vi "myXi_InitializeFreeRunnin.vi"(7 "subimage IN":refnum<vi>, 8 "error in (no error)":errorcluster, 11 "xiCam IN":refnum<k24>) -> (0 "error out":errorcluster, 2 "Array":u8[](array[numeric]), 3 "xiCam Out":refnum<k24>)   [LabVIEW 2018]
uses:
  C:/XIMEA/API/x64/xiApi.NETX64.dll
  VisionLibrariesXimea/xiLib/xiLIB_64bit/xiLIB/xiCamLib/xiCam/PRM/PRM/PRM_v2.ctl
  VisionLibrariesXimea/xiLib/xiLIB_64bit/xiLIB/xiCamLib/xiCam/PRM/TRG_SOURCE/TRG_SOURCE.ctl
  VisionLibrariesXimea/xiLib/xiLIB_64bit/xiLIB/xiCamLib/xiCam/PRM/TRG_SELECTOR/TRG_SELECTOR.ctl
  VisionLibrariesXimea/xiLib/xiLIB_64bit/xiLIB/xiCamLib/xiLIB/xiLIB - GetPRM_INFO.vi
  VisionLibrariesXimea/xiLib/xiLIB_64bit/xiLIB/xiCamLib/xiCam/Methods/xiCam - GetParam_Float.vi
  VisionLibrariesXimea/xiLib/xiLIB_64bit/xiLIB/xiCamLib/xiCam/Methods/xiCam - GetParam_String.vi
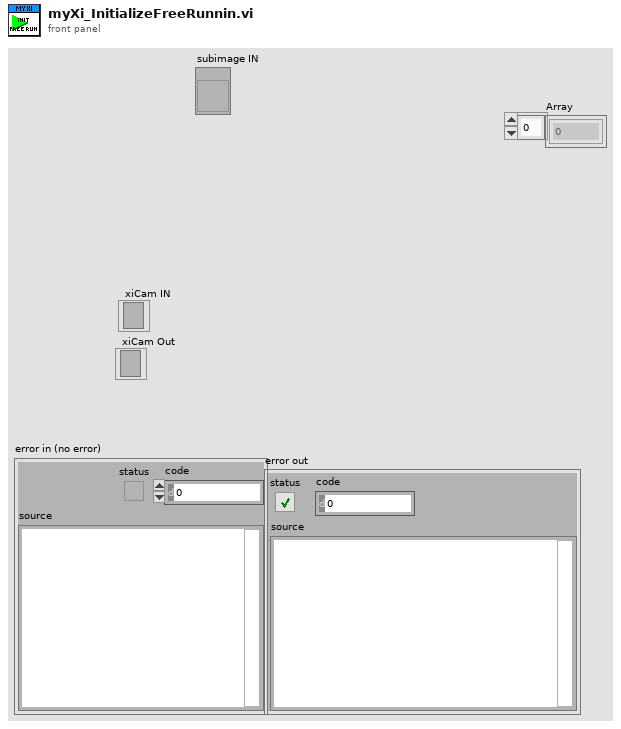
[diagram p1: front panel]
types:
  T1 = typedef "PRM_v2.ctl" = enum16{"ACQ_BUFFER_SIZE", "ACQ_FRAME_BURST_COUNT", "ACQ_TIMING_MODE", "ACQ_TRANSPORT_BUFFER_SIZE", "AE_MAX_LIMIT", "AEAG", "AEAG_LEVEL", "API_VERSION", "AG_MAX_LIMIT", "APPLY_CMS", "AUTO_BANDWIDTH_CALCULATION", "AUTO_WB", "AVAILABLE_BANDWIDTH", "AVAILABLE_BANDWIDTH_MAX", "AVAILABLE_BANDWIDTH_MIN", "BPC", "BUFFER_POLICY", "BUFFERS_QUEUE_SIZE", "CC_MATRIX_00", "CC_MATRIX_01", "CC_MATRIX_02", "CC_MATRIX_03", "CC_MATRIX_10", "CC_MATRIX_11", "CC_MATRIX_12", "CC_MATRIX_13", "CC_MATRIX_20", "CC_MATRIX_21", "CC_MATRIX_22", "CC_MATRIX_23", "CC_MATRIX_30", "CC_MATRIX_31", "CC_MATRIX_32", "CC_MATRIX_33", "CHIP_TEMP", "CMS", "COLOR_FILTER_ARRAY", "COOLING", "DEBOUNCE_EN", "DEBOUNCE_POL", "DEBOUNCE_T0", "DEBOUNCE_T1", "DEBUG_LEVEL", "DEFAULT_CC_MATRIX", "DEVICE_INSTANCE_PATH", "DEVICE_MODEL_ID", "DEVICE_NAME", "DEVICE_SN", "DEVICE_TYPE", "DEVICE_USER_ID", "DOWNSAMPLING", "DOWNSAMPLING_MAX", "DOWNSAMPLING_MIN", "DOWNSAMPLING_TYPE", "DRV_VERSION", "EXP_PRIORITY", "EXPOSURE", "EXPOSURE_DIRECT_UPDATE", "EXPOSURE_MAX", "EXPOSURE_MIN", "FFS_FILE_NAME", "FPGA1_VERSION", "FRAMERATE", "FRAMERATE_MAX", "FRAMERATE_MIN", "FREE_FFS_SIZE", "GAIN", "GAIN_DIRECT_UPDATE", "GAIN_MAX", "GAIN_MIN", "GAMMAC", "GAMMAY", "GPI_LEVEL", "GPI_MODE", "GPI_SELECTOR", "GPI_SELECTOR_MAX", "GPI_SELECTOR_MIN", "GPO_MODE", "GPO_SELECTOR", "GPO_SELECTOR_MAX", "GPO_SELECTOR_MIN", "HDR", "HDR_T1", "HDR_T2", "HEIGHT", "HEIGHT_MAX", "HEIGHT_MIN", "HOUSE_TEMP", "IMAGE_DATA_FORMAT", "IMAGE_IS_COLOR", "INPUT_CMS_PROFILE", "IS_COOLED", "IS_DEVICE_EXIST", "KNEEPOINT1", "KNEEPOINT2", "LED_MODE", "LED_SELECTOR", "LED_SELECTOR_MAX", "LED_SELECTOR_MIN", "LIMIT_BANDWIDTH", "LIMIT_BANDWIDTH_MAX", "LIMIT_BANDWIDTH_MIN", "LUT_EN", "LUT_INDEX", "LUT_INDEX_MAX", "LUT_INDEX_MIN", "LUT_VALUE", "LUT_VALUE_MAX", "LUT_VALUE_MIN", "MANUAL_WB", "MCU1_VERSION", "MCU2_VERSION", "OFFSET_X", "OFFSET_X_MAX", "OFFSET_X_MIN", "OFFSET_Y", "OFFSET_Y_MAX", "OFFSET_Y_MIN", "OUTPUT_CMS_PROFILE", "OUTPUT_DATA_BIT_DEPTH", "OUTPUT_DATA_PACKING", "READ_FILE_FFS", "RECENT_FRAME", "SENSOR_DATA_BIT_DEPTH", "SENSOR_MODE", "SENSOR_TAPS", "SHARPNESS", "SHUTTER_TYPE", "TARGET_TEMP", "TRG_DELAY", "TRG_SELECTOR", "TRG_SOFTWARE", "TRG_SOURCE", "USED_FFS_SIZE", "WB_KB", "WB_KG", "WB_KR", "WIDTH", "WIDTH_MAX", "WIDTH_MIN", "WRITE_FILE_FFS", "ACQ_BUFFER_SIZE_UNIT", "ACQ_TRANSPORT_BUFFER_COMMIT", "AEAG_ROI_HEIGHT", "AEAG_ROI_OFFSET_X", "AEAG_ROU_OFFSET_Y", "AEAG_ROI_WIDTH", "API_CONTEXT_LIST", "BINNING_HORIZONTAL", "BINNING_SELECTOR", "BINNING_VERTICAL", "COLUMN_FPN_CORRECTION", "COUNTER_SELECTOR", "COUNTER_VALUE", "DECIMATION_HORIZONTAL", "DECIMATION_SELECTOR", "DECIMATION_VERTICAL", "DEVICE_ID", "DEVICE_LOCATION_PATH", "DEVICE_MANIFEST", "DEVICE_RESET", "DEVICE_SENS_SN", "EXPOSURE_BURST_COUNT", "FFS_ACCESS_KEY", "GAIN_SELECTOR", "HW_REVISION", "IMAGE_BLACK_LEVEL", "IMAGE_DATA_BIT_DEPTH", "IMAGE_DATA_FORMAT_RGB32_ALPHA", "IMAGE_PAYLOAD_SIZE", "LENS_APERTURE_VALUE", "LENS_FEATURE", "LENS_FEATURE_SELECTOR", "LENS_FOCAL_LENGTH", "LENS_FOCUS_DISTANCE", "LENS_FOCUS_MOVE", "LENS_FOCUS_MOVEMENT_VALUE", "LENS_MODE", "OUTPUT_DATA_PACKING_TYPE", "SENSOR_CLOCK_FREQ_HZ", "SENSOR_CLOCK_FREQ_INDEX", "SENSOR_FEATURE_SELECTOR", "SENSOR_FEATURE_VALUE", "SENSOR_OUTPUT_CHANNEL_COUNT", "TRANSPORT_PIXEL_FORMAT", "TS_RST_MODE", "TS_RST_SOURCE"}
  T2 = typedef "TRG_SOURCE.ctl" = enum16{"OFF", "EDGE_RISING", "EDGE_FALLING", "SOFTWARE"}
  T3 = typedef "TRG_SELECTOR.ctl" = enum16{"FRAME_START", "EXPOSURE_ACTIVE", "FRAME_BURST_START", "FRAME_BURST_ACTIVE"}
  T4 = typedef "LVPointDoubleTypeDef.ctl" = cluster{"X":dbl, "Y":dbl}
  T5 = cluster{"2^n : x":i8, "2^n : y":i8, "lower left box Position":T4, "Height":i32, "Width":i32}
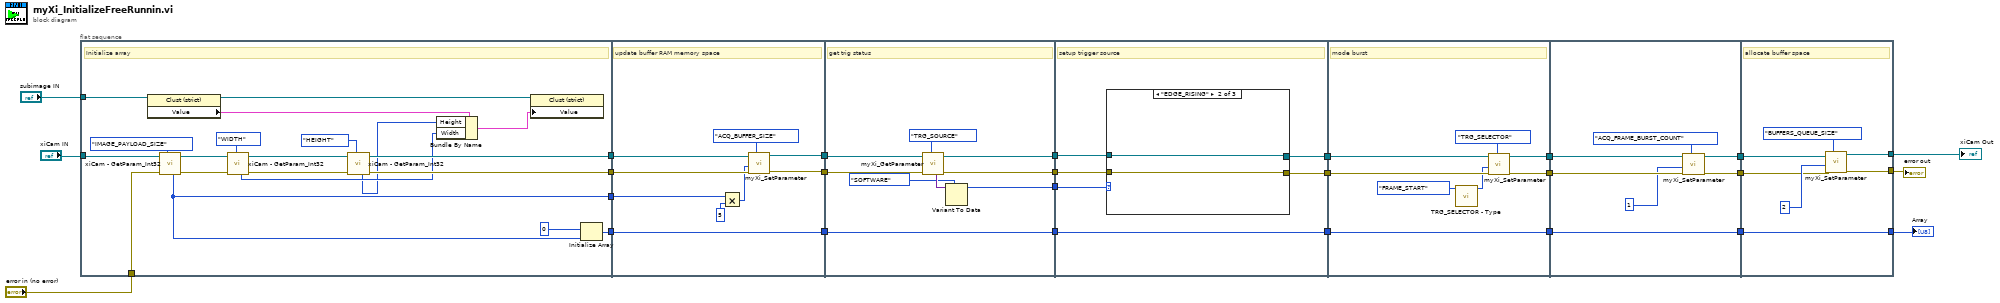
[diagram p0: block diagram]
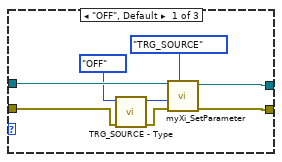
[diagram p2: hidden frame]
diagram:
  n1 = flat-sequence {
    tunnel: "xiCam IN" -> [w46]
    tunnel: [w43] -> w26
    tunnel: "error in (no error)" -> [w42]
    tunnel: [w41] -> w25
    tunnel: [w39] -> w24
    tunnel: "subimage IN" -> [w38]
    tunnel: [w27] -> w1
    tunnel: w26 -> [w53]
    tunnel: [w52] -> w23
    tunnel: w25 -> [w55]
    tunnel: [w54] -> w22
    tunnel: w24 -> [w50]
    tunnel: [w50] -> w21
    tunnel: w1 -> [w47]
    tunnel: w23 -> [w61]
    tunnel: [w60] -> w20
    tunnel: w22 -> [w63]
    tunnel: [w62] -> w19
    tunnel: w21 -> [w64]
    tunnel: [w64] -> w18
    tunnel: [w56] -> w17
    tunnel: [w69] -> w16
    tunnel: [w68] -> w15
    tunnel: w20 -> [w70]
    tunnel: w19 -> [w67]
    tunnel: [w66] -> w14
    tunnel: w18 -> [w66]
    tunnel: w17 -> [w65]
    tunnel: w16 -> [w89]
    tunnel: w15 -> [w88]
    tunnel: w14 -> [w83]
    tunnel: [w85] -> w8
    tunnel: [w84] -> w6
    tunnel: [w83] -> w4
    tunnel: w8 -> [w95]
    tunnel: [w94] -> w7
    tunnel: w6 -> [w93]
    tunnel: [w92] -> w5
    tunnel: w4 -> [w97]
    tunnel: [w97] -> w3
    tunnel: [w103] -> w11
    tunnel: [w102] -> w12
    tunnel: w7 -> [w100]
    tunnel: w5 -> [w99]
    tunnel: [w98] -> w9
    tunnel: w3 -> [w98]
    frame #0 {
      # "Initialize array"
      n2 = property class="Clust (strict)"(reference=w38) -> (reference out=w37:refnum<vi>, "Value"=w36:T5)  [unwired: 1 in, 1 out]
      n3 = call "xiCam - GetParam_Int32.vi"("PRM"=PRM_v2."IMAGE_PAYLOAD_SIZE", "error in (no error)"=w42, "xiCam In"=w46) -> ("error out"=w34:errorcluster, "xiCam Out"=w32:refnum<k24>, "Int32_Value"=w27:i32)  [unwired: 6 in]
      n4 = call "xiCam - GetParam_Int32.vi"("PRM"=PRM_v2."WIDTH", "error in (no error)"=w34, "xiCam In"=w32) -> ("error out"=w33:errorcluster, "xiCam Out"=w31:refnum<k24>, "Int32_Value"=w29:i32)  [unwired: 6 in]
      n5 = call "xiCam - GetParam_Int32.vi"("PRM"=PRM_v2."HEIGHT", "error in (no error)"=w33, "xiCam In"=w31) -> ("error out"=w41:errorcluster, "xiCam Out"=w43:refnum<k24>, "Int32_Value"=w28:i32)  [unwired: 6 in]
      n6 = Bundle By Name(cluster=w36, "Height"=w28, "Width"=w29) -> (w35:T5)
      n7 = property class="Clust (strict)"(reference=w37, "Value"=w35) -> ()  [unwired: 1 in, 2 out]
      n8 = Initialize Array "Initialize Array"(u8 0 ("element"), w27) -> (w39:u8[])
    }
    frame #1 {
      # "update buffer RAM memory space"
      n9 = Multiply(x=w47, y=i64 5 ("image frames")) -> (x*y=w49:i64)
      n10 = call "myXi_SetParameter.vi"("input PRM"=PRM_v2."ACQ_BUFFER_SIZE", "error in"=w55, "input value I32"=w49, "xiCam IN"=w53) -> ("error out"=w54:errorcluster, "xiCam Out"=w52:refnum<k24>)  [unwired: 6 in]
    }
    frame #2 {
      # "get trig status"
      n11 = call "myXi_GetParameter.vi"("input PRM"=PRM_v2."TRG_SOURCE", "error in"=w63, "xiCam IN"=w61) -> ("error out"=w62:errorcluster, "xiCam Out"=w60:refnum<k24>, "output"=w58:variant)  [unwired: 3 in, 3 out]
      n12 = Variant To Data(type=TRG_SOURCE."SOFTWARE" ("TRG_SOURCE"), Variant=w58) -> (data=w56:T2)  [unwired: 1 in, 1 out]
    }
    frame #3 {
      # "setup trigger source"
      n13 = case shown="\"EDGE_RISING\"" w65 {
        tunnel: w70 -> [w78 w80 w82]
        tunnel: [w77 w79 w81] -> w69
        tunnel: [w76 w80 w82] -> w68
        tunnel: w67 -> [w75 w79 w81]
        frame "OFF", Default {
          n14 = call "TRG_SOURCE - Type.vi"("error in (no error)"=w75, "TRG_SOURCE"=TRG_SOURCE."OFF") -> ("error out"=w72:errorcluster, "TRG_SOURCE_VALUE"=w73:i32)  [unwired: 8 in]
          n15 = call "myXi_SetParameter.vi"("input PRM"=PRM_v2."TRG_SOURCE", "error in"=w72, "input value I32"=w73, "xiCam IN"=w78) -> ("error out"=w77:errorcluster, "xiCam Out"=w76:refnum<k24>)  [unwired: 6 in]
        }
        frame "EDGE_RISING" {
        }
        frame "EDGE_FALLING" {
        }
      }
    }
    frame #4 {
      # "mode burst"
      n16 = call "TRG_SELECTOR - Type.vi"("TRG_SELECTOR"=TRG_SELECTOR."FRAME_START") -> ("TRG_SELECTOR_VALUE"=w86:i32)  [unwired: 9 in, 1 out]
      n17 = call "myXi_SetParameter.vi"("input PRM"=PRM_v2."TRG_SELECTOR", "error in"=w89, "input value I32"=w86, "xiCam IN"=w88) -> ("error out"=w85:errorcluster, "xiCam Out"=w84:refnum<k24>)  [unwired: 6 in]
    }
    frame #5 {
      n18 = call "myXi_SetParameter.vi"("input PRM"=PRM_v2."ACQ_FRAME_BURST_COUNT", "error in"=w95, "input value I32"=i64 1, "xiCam IN"=w93) -> ("error out"=w94:errorcluster, "xiCam Out"=w92:refnum<k24>)  [unwired: 6 in]
    }
    frame #6 {
      # "allocate buffer space"
      n19 = call "myXi_SetParameter.vi"("input PRM"=PRM_v2."BUFFERS_QUEUE_SIZE", "error in"=w100, "input value I32"=i64 2, "xiCam IN"=w99) -> ("error out"=w103:errorcluster, "xiCam Out"=w102:refnum<k24>)  [unwired: 6 in]
    }
  }
  "xiCam Out" <- w12
  "error out" <- w11
  "Array" <- w9
